vi "Write Name.vi"(8 "error in (no error)":errorcluster, 10 "Name":string, 11 "Chat Window UI Controller in":refnum<class "Chat Window UI Controller.lvclass">) -> (0 "error out":errorcluster, 3 "Chat Window UI Controller out":refnum<class "Chat Window UI Controller.lvclass">)   [LabVIEW 2019, in "Chat Window UI Controller.lvlib" / "Chat Window UI Controller.lvclass"]
uses:
  Chat Window UI Controller.lvclass
  Chat Window UI Controller.lvclass/Chat Window UI Controller.ctl
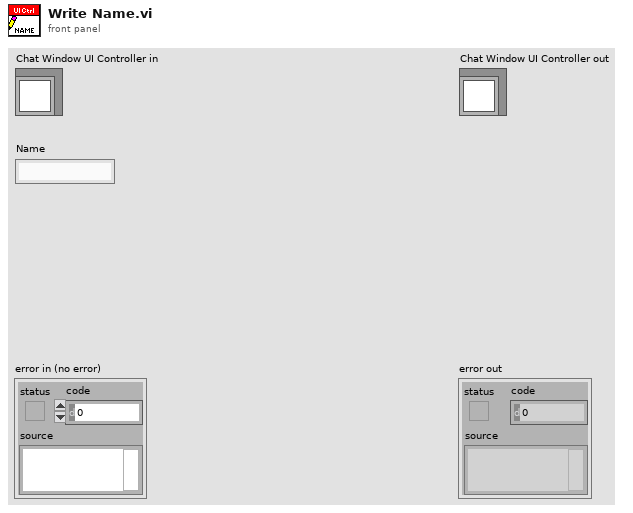
[diagram p1: front panel]
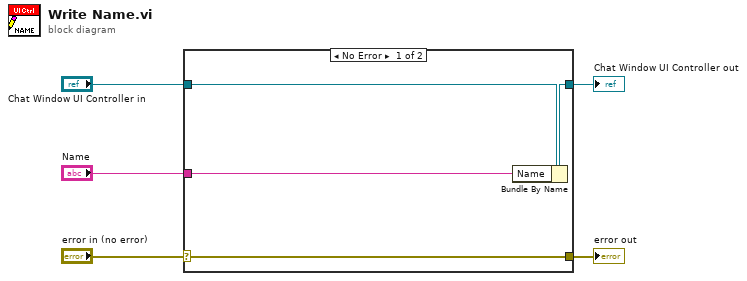
[diagram p0: block diagram]
diagram:
  n1 = case shown="No Error" "error in (no error)" {
    selector: "error in (no error)" -> [w9 w10]
    tunnel: [w9 w10] -> w4
    tunnel: [w7 w11] -> w2
    tunnel: "Chat Window UI Controller in" -> [w8 w11]
    tunnel: "Name" -> [w6 _]
    frame No Error {
      n2 = Bundle By Name(cluster=w8, "Name"=w6) -> (w7:refnum<class "Chat Window UI Controller.lvclass">)
    }
    frame Error {
    }
  }
  "error out" <- w4
  "Chat Window UI Controller out" <- w2
